vi "Dynamixel Motor Setup.vi"() -> ()   [LabVIEW 2016]
doc: "This example is designed for configuring attributes typically set on a dynamixel motor before first use."
uses:
  <instrlib>/Dynamixel Motor/Public/Motor Operation/Low Level/Alarm Setting.ctl
  <instrlib>/Dynamixel Motor/Public/Motor Operation/Low Level/Baud Setting.ctl
  <instrlib>/Dynamixel Motor/HAIOL/Dynamixel Motor.lvclass
  <instrlib>/Dynamixel Motor/HAIOL/VISA/Dynamixel Motor VISA.lvclass
  <instrlib>/Dynamixel Motor/Dynamixel Motor.lvlib
panel:
  out "Searching for motor":bool
  in  "Tab Control":enum32{"Port setup", "Auto-detect settings"}(tab)
  in  "VISA resource name":refnum<visa-resource-name>
  in  "Baud rate (57600 bps)":T1=34 items=["1,000,000 bps"=1, "500,000 bps"=3, "400,000 bps"=4, "250,000 bps"=7, "200,000 bps"=9, "115200 bps"=16, "57600 bps"=34, "19200 bps"=103, "9600 bps"=207]
  in  "Force Baud Rate (True)":bool=TRUE
  in  "Search Timeout (10000 ms)":u32=10000
  in  "Starting ID (0)":u8
  in  "Ending ID (253)":u8=253
  in  "stop":bool
  out "Current angles":cluster{dbl, dbl, dbl}(knob)={0.0, 0.0, 300.0} scale=0.0..300.0
  in  "Counter-Clockwise Limit":dbl=300.0
  in  "Clockwise Limit":dbl
  out "Current Safety Limits":T2={"Temperature Limit (C)"=80, "Low Voltage Limit (V)"=6.0, "High Voltage Limit (V)"=19.0, "Maximum Torque%"=100.0} {"Maximum Torque%" min=0.0 max=100.0; "High Voltage Limit (V)" min=5.0 max=25.0; "Low Voltage Limit (V)" min=5.0 max=25.0; "Temperature Limit (C)" max=150 step=1}
  in  "Desired Safety Limits":T2={"Temperature Limit (C)"=80, "Low Voltage Limit (V)"=6.0, "High Voltage Limit (V)"=19.0, "Maximum Torque%"=100.0} {"Maximum Torque%" min=0.0 max=100.0; "High Voltage Limit (V)" min=5.0 max=25.0; "Low Voltage Limit (V)" min=5.0 max=25.0; "Temperature Limit (C)" max=150 step=1}
  in  "Apply new settings":bool
  out "Current Alarm Settings":cluster{"LED Alarm":T3, "Shutdown Alarm":T3}={"LED Alarm"={"Input Voltage"=FALSE, "Angle Limit"=FALSE, "Overheating "=TRUE, "Range"=FALSE, "Checksum"=FALSE, "Overload"=TRUE, "Instruction"=FALSE}, "Shutdown Alarm"={"Input Voltage"=FALSE, "Angle Limit"=FALSE, "Overheating "=TRUE, "Range"=FALSE, "Checksum"=FALSE, "Overload"=TRUE, "Instruction"=FALSE}}
  in  "Desired Alarm Settings":cluster{"LED Alarm":T3, "Shutdown Alarm":T3}={"LED Alarm"={"Input Voltage"=FALSE, "Angle Limit"=FALSE, "Overheating "=TRUE, "Range"=FALSE, "Checksum"=FALSE, "Overload"=TRUE, "Instruction"=FALSE}, "Shutdown Alarm"={"Input Voltage"=FALSE, "Angle Limit"=FALSE, "Overheating "=TRUE, "Range"=FALSE, "Checksum"=FALSE, "Overload"=TRUE, "Instruction"=FALSE}}
  in  "Change ID":bool
  out "Current ID":u8
  in  "New ID":u8
  # "(c) 2011  National Instruments.  ALL RIGHTS RESERVED."
  # "This example is designed for \nconfiguring attributes typically set \non a Dynamixel motor before first \nuse.  \n\n1. Connect only one motor to the\nserial communications line. \n2. Choose the serial communication \nsettings and optionally the auto \ndetect settings.  \n3. Run the VI.\n4. Change the ID if desired.\n5. Enter other desired settings and\nclick Apply new settings.\n6. Stop the VI and repeat for each\nmotor you wish to configure."
  # "Clockwise Limit"
  # "Motor Position"
  # "Counter-Clockwise Limit"
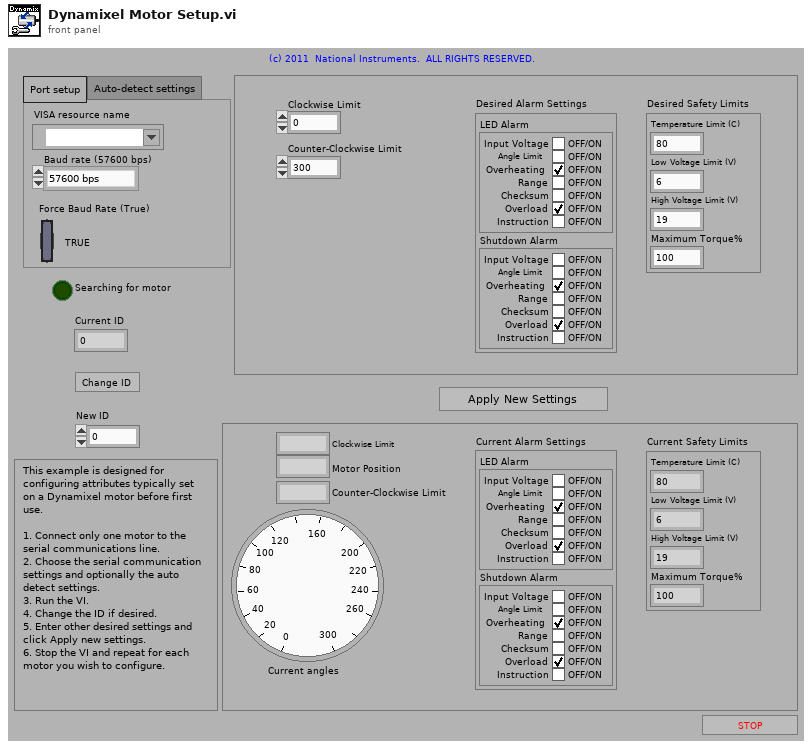
[diagram p1: front panel]
types:
  T1 = typedef "Dynamixel Motor.lvlib/Baud Setting.ctl" = u8
  T2 = cluster{"Temperature Limit (C)":u8, "Low Voltage Limit (V)":dbl, "High Voltage Limit (V)":dbl, "Maximum Torque%":dbl}
  T3 = typedef "Dynamixel Motor.lvlib/Alarm Setting.ctl" = cluster{"Input Voltage":bool, "Angle Limit":bool, "Overheating ":bool, "Range":bool, "Checksum":bool, "Overload":bool, "Instruction":bool}
  T4 = cluster{"Boolean array[0]":bool, "Boolean array[1]":bool, "Boolean array[2]":bool, "Boolean array[3]":bool, "Boolean array[4]":bool, "Boolean array[5]":bool, "Boolean array[6]":bool}
  T5 = cluster{"Boolean array":cluster{"Boolean array[0]":bool, "Boolean array[1]":bool, "Boolean array[2]":bool, "Boolean array[3]":bool, "Boolean array[4]":bool, "Boolean array[5]":bool, "Boolean array[6]":bool}, "Boolean array":cluster{"Boolean array[0]":bool, "Boolean array[1]":bool, "Boolean array[2]":bool, "Boolean array[3]":bool, "Boolean array[4]":bool, "Boolean array[5]":bool, "Boolean array[6]":bool}}
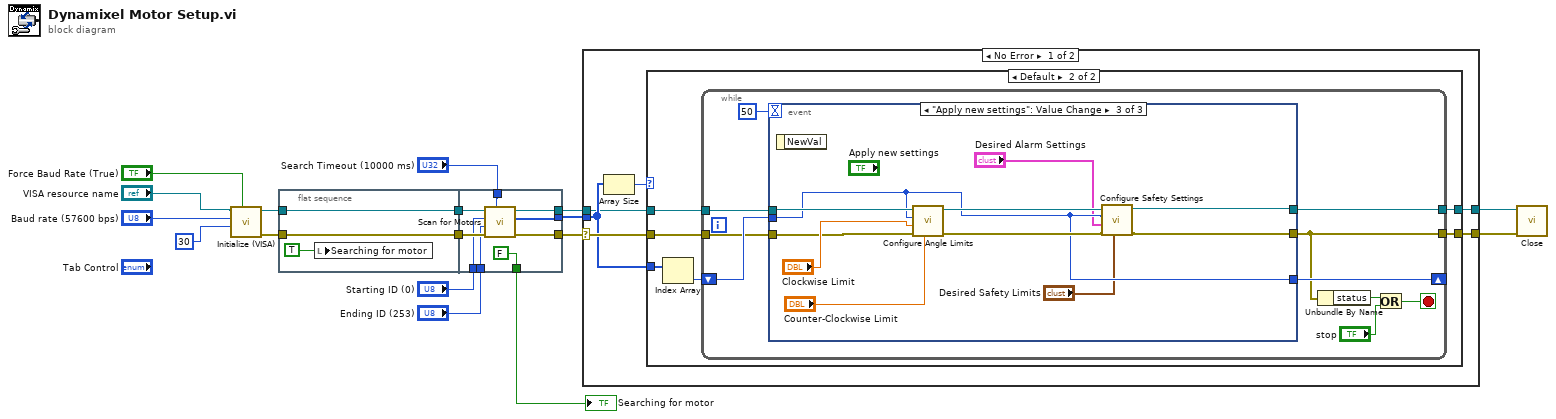
[diagram p0: block diagram]
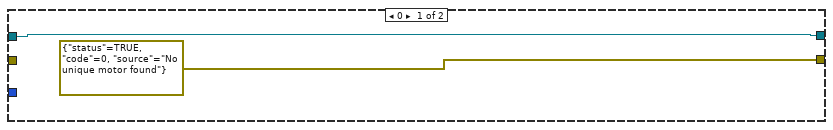
[diagram p2: hidden frame]
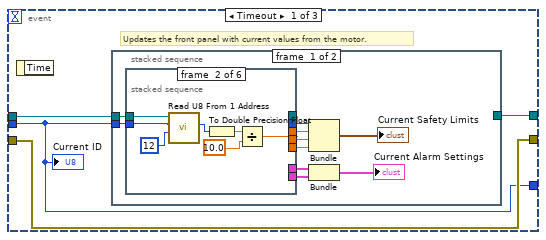
[diagram p3: hidden frame]
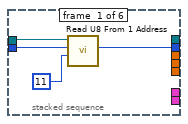
[diagram p4: hidden frame]
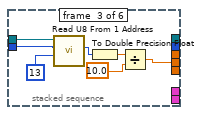
[diagram p5: hidden frame]
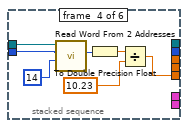
[diagram p6: hidden frame]
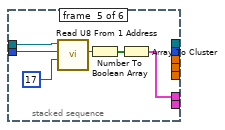
[diagram p7: hidden frame]
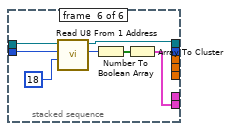
[diagram p8: hidden frame]
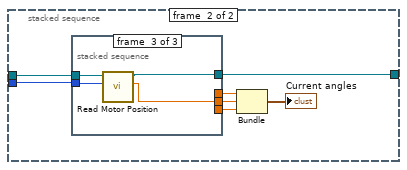
[diagram p9: hidden frame]
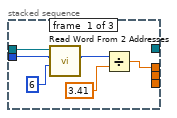
[diagram p10: hidden frame]
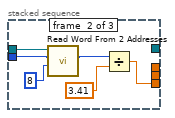
[diagram p11: hidden frame]
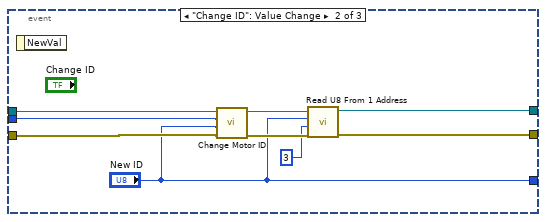
[diagram p12: hidden frame]
diagram:
  n1 = call <instrlib>:"Initialize (VISA).vi"("Force Baud Rate (True)"="Force Baud Rate (True)", "Timeout (30 msec)"=u32 30 ("timeout (10sec)"), "Baud rate (57600 bps)"="Baud rate (57600 bps)", "VISA resource name"="VISA resource name") -> ("error out"=w6:errorcluster, "Dynamixel Motor out"=w7:refnum<class "Dynamixel Motor.lvclass">)  [unwired: 6 in]
  n2 = flat-sequence {
    tunnel: w7 -> [w19]
    tunnel: w6 -> [w18]
    tunnel: [w19] -> w5
    tunnel: [w18] -> w4
    tunnel: [w21] -> w17
    tunnel: [w22] -> w16
    tunnel: "Search Timeout (10000 ms)" -> [w28]
    tunnel: "Starting ID (0)" -> [w25]
    tunnel: "Ending ID (253)" -> [w24]
    tunnel: [FALSE ("Searching for motor")] -> w12
    tunnel: w5 -> [w27]
    tunnel: w4 -> [w26]
    tunnel: [w23] -> w3
    frame #0 {
      n3 = local write "Searching for motor"(TRUE ("Searching for motor")) -> ()
    }
    frame #1 {
      n4 = call-dynamic "Scan for Motors.vi"("Search Timeout (10000 ms)"=w28, "error in (no error)"=w26, "Ending ID (253)"=w24, "Starting ID (0)"=w25, "Dynamixel Motor in"=w27) -> ("error out"=w21:errorcluster, "Motors IDs Found"=w22:u8[], "Dynamixel Motor out"=w23:refnum<class "Dynamixel Motor.lvclass">)  [unwired: 4 in]
    }
  }
  n5 = case shown="No Error" w17 {
    selector: w17 -> [w35 w150]
    tunnel: [w34 w150] -> w1
    tunnel: w16 -> [w33 _]
    tunnel: w3 -> [w31 w149]
    tunnel: [w30 w149] -> w2
    frame No Error {
      n6 = Array Size(array=w33) -> (size(s)=w32:i32)
      n7 = case shown="Default" w32 {
        tunnel: w35 -> [_ w43]
        tunnel: w33 -> [_ w42]
        tunnel: [errorcluster {"status"=TRUE, "code"=0, "source"="No unique motor found"} ("error out") w40] -> w34
        tunnel: w31 -> [w36 w39]
        tunnel: [w36 w38] -> w30
        frame 0 {
        }
        frame Default {
          n8 = Index Array(array=w42) -> (element=w41:u8)  [unwired: 1 in]
          n9 = while {
            tunnel: w43 -> [w50]
            shift-right: [w49] -> _
            shift-left: w41 -> [w52]
            tunnel: [w51] -> w38
            tunnel: [w48] -> w40
            tunnel: w39 -> [w44]
            stop <- w47 stop-if-true
            n10 = event shown="[2] \"Apply new settings\": Value Change" {
              selector: _ -> [_ _ _]
              dyn-events: _ -> [_ _ _]
              timeout: 50 -> [_ _ _]
              tunnel: w52 -> [w55 w136 w141]
              tunnel: [w57 w129 w138] -> w51
              tunnel: w50 -> [w56 w135 w145]
              tunnel: [w56 w130 w144] -> w48
              tunnel: [w55 "New ID" w141] -> w49
              tunnel: w44 -> [w54 w137 w148]
              event Timeout {
                # "Updates the front panel with current values from the motor."
                n11 = event-data() -> ()  [unwired: 1 in, 1 out]
                n12 = stacked-sequence {
                  tunnel: w55 -> [w59 w108]
                  tunnel: [_ w107] -> w57
                  tunnel: w54 -> [w58 w106]
                  frame #0 {
                    n13 = stacked-sequence {
                      tunnel: [w68 _ _ _ _ _] -> w65
                      tunnel: [_ w76 _ _ _ _] -> w64
                      tunnel: [_ _ w83 _ _ _] -> w63
                      tunnel: [_ _ _ w90 _ _] -> w62
                      tunnel: [_ _ _ _ w97 _] -> w61
                      tunnel: [_ _ _ _ _ w104] -> w60
                      tunnel: w59 -> [w70 w74 w81 w88 w95 w102]
                      tunnel: w58 -> [w71 w75 w82 w89 w96 w103]
                      tunnel: [_ _ _ _ _ w99] -> _
                      frame #0 {
                        n14 = call-dynamic "Read U8 From 1 Address.vi"("Address number (0)"=u8 11 ("Address # DEC"), "Motor ID (0)"=w70, "Dynamixel Motor in"=w71) -> ("Data"=w68:u8)  [unwired: 6 in, 2 out]
                      }
                      frame #1 {
                        n15 = call-dynamic "Read U8 From 1 Address.vi"("Address number (0)"=u8 12 ("Address # DEC"), "Motor ID (0)"=w74, "Dynamixel Motor in"=w75) -> ("Data"=w72:u8)  [unwired: 6 in, 2 out]
                        n16 = To Double Precision Float(number=w72) -> (double precision float=w78:dbl)
                        n17 = Divide(x=w78, y=10.0) -> (x/y=w76:dbl)
                      }
                      frame #2 {
                        n18 = call-dynamic "Read U8 From 1 Address.vi"("Address number (0)"=u8 13 ("Address # DEC"), "Motor ID (0)"=w81, "Dynamixel Motor in"=w82) -> ("Data"=w79:u8)  [unwired: 6 in, 2 out]
                        n19 = To Double Precision Float(number=w79) -> (double precision float=w85:dbl)
                        n20 = Divide(x=w85, y=10.0) -> (x/y=w83:dbl)
                      }
                      frame #3 {
                        n21 = call-dynamic "Read Word From 2 Addresses.vi"("Address number (0)"=u8 14 ("Address # DEC"), "Motor ID (0)"=w88, "Dynamixel Motor in"=w89) -> ("Data"=w86:u8)  [unwired: 6 in, 2 out]
                        n22 = To Double Precision Float(number=w86) -> (double precision float=w92:dbl)
                        n23 = Divide(x=w92, y=10.23) -> (x/y=w90:dbl)
                      }
                      frame #4 {
                        n24 = call-dynamic "Read U8 From 1 Address.vi"("Address number (0)"=u8 17 ("Address # DEC"), "Motor ID (0)"=w95, "Dynamixel Motor in"=w96) -> ("Data"=w93:u8)  [unwired: 6 in, 2 out]
                        n25 = Number To Boolean Array(number=w93) -> (Boolean array=w98:bool[])
                        n26 = Array To Cluster(array=w98) -> (cluster=w97:T4)
                      }
                      frame #5 {
                        n27 = call-dynamic "Read U8 From 1 Address.vi"("Address number (0)"=u8 18 ("Address # DEC"), "Motor ID (0)"=w102, "Dynamixel Motor in"=w103) -> ("Data"=w100:u8, "Dynamixel Motor out"=w99:refnum<class "Dynamixel Motor.lvclass">)  [unwired: 6 in, 1 out]
                        n28 = Number To Boolean Array(number=w100) -> (Boolean array=w105:bool[])
                        n29 = Array To Cluster(array=w105) -> (cluster=w104:T4)
                      }
                    }
                    n30 = Bundle("Data"=w65, w64, w63, w62) -> (→"Current Safety Limits":cluster{"Data":u8, dbl, dbl, dbl})  [unwired: 1 in]
                    n31 = Bundle("Boolean array"=w61, "Boolean array"=w60) -> (→"Current Alarm Settings":T5)  [unwired: 1 in]
                  }
                  frame #1 {
                    n32 = stacked-sequence {
                      tunnel: w108 -> [w116 w121 w127]
                      tunnel: [w117 _ _] -> w111
                      tunnel: [_ _ w125] -> w110
                      tunnel: [_ w123 _] -> w109
                      tunnel: [_ _ w126] -> w107
                      tunnel: w106 -> [w113 w122 w128]
                      frame #0 {
                        n33 = call-dynamic "Read Word From 2 Addresses.vi"("Address number (0)"=u8 6 ("Address # DEC"), "Motor ID (0)"=w116, "Dynamixel Motor in"=w113) -> ("Data"=w115:u8)  [unwired: 6 in, 2 out]
                        n34 = Divide(x=w115, y=3.41) -> (x/y=w117:dbl)
                      }
                      frame #1 {
                        n35 = call-dynamic "Read Word From 2 Addresses.vi"("Address number (0)"=u8 8 ("Address # DEC"), "Motor ID (0)"=w121, "Dynamixel Motor in"=w122) -> ("Data"=w119:u8)  [unwired: 6 in, 2 out]
                        n36 = Divide(x=w119, y=3.41) -> (x/y=w123:dbl)
                      }
                      frame #2 {
                        n37 = call-dynamic "Read Motor Position.vi"("Motor ID (0)"=w127, "Dynamixel Motor in"=w128) -> ("Position (deg)"=w125:dbl, "Dynamixel Motor out"=w126:refnum<class "Dynamixel Motor.lvclass">)  [unwired: 7 in, 1 out]
                      }
                    }
                    n38 = Bundle(w111, "Position (deg)"=w110, w109) -> (→"Current angles":cluster{dbl, "Position (deg)":dbl, dbl})  [unwired: 1 in]
                  }
                }
                "Current ID" <- w55
              }
              event "Change ID": Value Change {
                n39 = event-data() -> ()  [unwired: 1 in, 1 out]
                n40 = call-dynamic "Change Motor ID.vi"("error in (no error)"=w135, "New ID"="New ID", "Current ID"=w136, "Dynamixel Motor in"=w137) -> ("error out"=w133:errorcluster, "Dynamixel Motor out"=w134:refnum<class "Dynamixel Motor.lvclass">)  [unwired: 6 in]
                n41 = call-dynamic "Read U8 From 1 Address.vi"("error in (no error)"=w133, "Address number (0)"=u8 3 ("Address number (dec)"), "Motor ID (0)"="New ID", "Dynamixel Motor in"=w134) -> ("error out"=w130:errorcluster, "Dynamixel Motor out"=w129:refnum<class "Dynamixel Motor.lvclass">)  [unwired: 5 in, 1 out]
              }
              event "Apply new settings": Value Change {
                n42 = event-data() -> ()  [unwired: 1 in, 1 out]
                n43 = call-dynamic "Configure Angle Limits.vi"("Counter-Clockwise Angle Limit (300 deg)"="Counter-Clockwise Limit", "error in (no error)"=w145, "Clockwise Angle Limit (0 deg)"="Clockwise Limit", "Motor ID (0)"=w141, "Dynamixel Motor in"=w148) -> ("error out"=w143:errorcluster, "Dynamixel Motor out"=w142:refnum<class "Dynamixel Motor.lvclass">)  [unwired: 5 in]
                n44 = call-dynamic "Configure Safety Settings.vi"("Safety Limits"="Desired Safety Limits", "error in (no error)"=w143, "Alarm Settings"="Desired Alarm Settings", "Motor ID (0)"=w141, "Dynamixel Motor in"=w142) -> ("error out"=w144:errorcluster, "Dynamixel Motor out"=w138:refnum<class "Dynamixel Motor.lvclass">)  [unwired: 5 in]
              }
            }
            n45 = Unbundle By Name(w48) -> ("status"=w46:bool)
            n46 = Or(x=w46, y="stop") -> (x .or. y?=w47:bool)
          }
        }
      }
    }
    frame Error {
    }
  }
  n47 = call-dynamic "Close.vi"("error in (no error)"=w1, "Dynamixel Motor in"=w2) -> ()  [unwired: 9 in, 1 out]
  "Searching for motor" <- w12
